vi "Test XYZ Table Stage Module All Axis.vi"() -> ()   [LabVIEW 2018]
uses:
  Hardware Mfg/Thorlabs Translation Stages/Controls/Translation Stage Cluster.ctl
  General/Controls/Translation Stage Types.ctl
  General/Controls/Translation Stage Parameters.ctl
  General/Controls/Set Get Controls.ctl
  Hardware Mfg/Thorlabs Translation Stages/Controls/Motion Translation Module Control2.ctl
panel:
  in  "Table Stages":T1={"X Stage"={"Position"=0.0, "Is.Enabled?"=FALSE, "Is.Connected?"=FALSE, "Device SN"="45876425", "AccelerationMaximum"=0.0, "VelocityMaximum"=0.0, "Acceleration"=0.0, "Velocity"=0.0, "waitTimeout (ms)"=0, "Model"=enum."Thorlabs LTS", "Is.Homed?"=FALSE}, "Y Stage"={"Position"=0.0, "Is.Enabled?"=FALSE, "Is.Connected?"=FALSE, "Device SN"="45995820", "AccelerationMaximum"=0.0, "VelocityMaximum"=0.0, "Acceleration"=0.0, "Velocity"=0.0, "waitTimeout (ms)"=0, "Model"=enum."Thorlabs LTS", "Is.Homed?"=FALSE}, "Z Stage"={"Position"=0.0, "Is.Enabled?"=FALSE, "Is.Connected?"=FALSE, "Device SN"="49107444", "AccelerationMaximum"=0.0, "VelocityMaximum"=0.0, "Acceleration"=0.0, "Velocity"=0.0, "waitTimeout (ms)"=0, "Model"=enum."Thorlabs MLJ", "Is.Homed?"=FALSE}}
  out "Cluster":T4
  in  "Z Pos":dbl caption="Position"
  in  "Y Pos":dbl caption="Position"
  in  "X Pos":dbl caption="Position"
  out "Error Out":errorcluster
  in  "Uninit":bool
  in  "Init":bool
  in  "Cancel Button":bool
  in  "Position":bool
  in  "Stop":bool
  in  "Home":bool
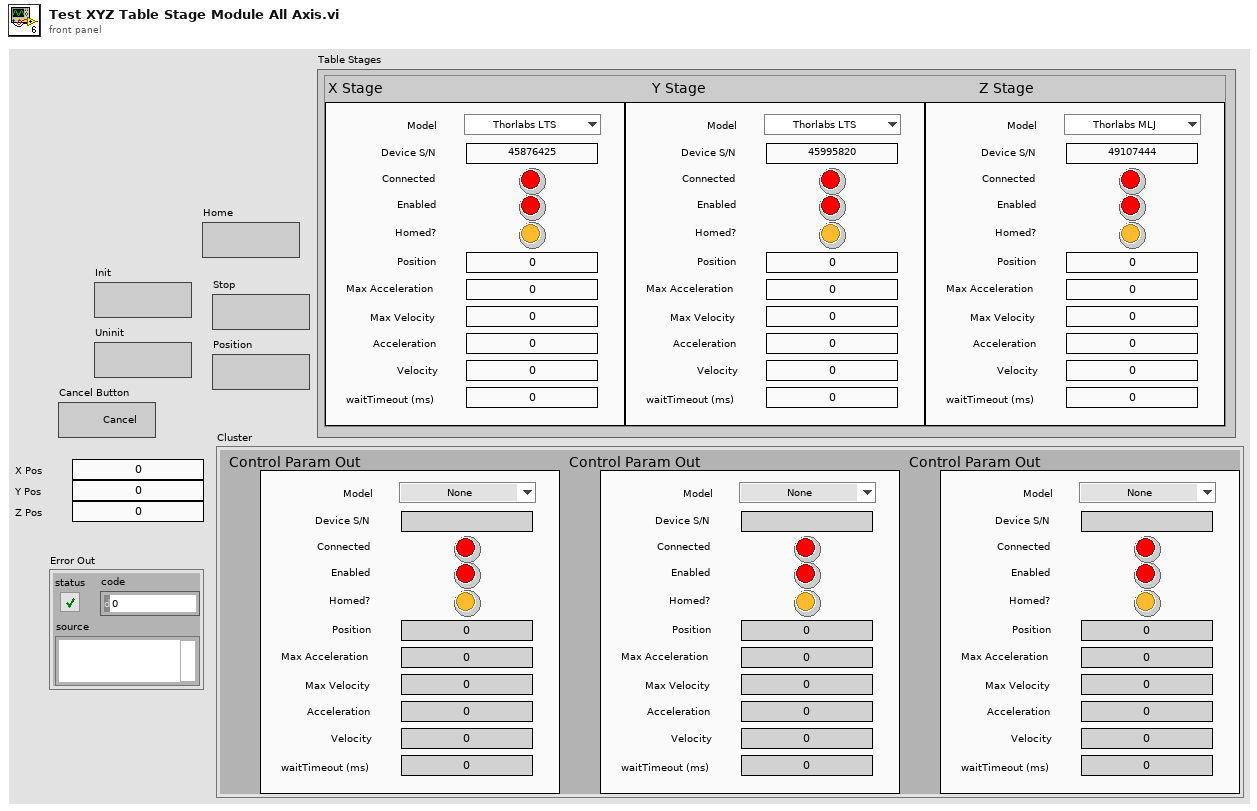
[diagram p1: front panel]
types:
  T1 = typedef "Translation Stage Parameters.ctl" = cluster{"X Stage":T2, "Y Stage":T2, "Z Stage":T2}
  T2 = typedef "Translation Stage Cluster.ctl" = cluster{"Position":dbl, "Is.Enabled?":bool, "Is.Connected?":bool, "Device SN":string, "AccelerationMaximum":dbl, "VelocityMaximum":dbl, "Acceleration":dbl, "Velocity":dbl, "waitTimeout (ms)":i32, "Model":T3, "Is.Homed?":bool}
  T3 = typedef "Translation Stage Types.ctl" = enum16{"None", "Thorlabs LTS", "Thorlabs MLJ"}
  T4 = cluster{"Control Param Out":T2, "Control Param Out":T2, "Control Param Out":T2}
  T5 = typedef "Motion Translation Module Control2.ctl" = enum16{"Init", "Home", "Status", "Velocity/Accel", "Position", "Jog", "Stop", "Uninit", "Enable", "Disable"}
  T6 = typedef "Set Get Controls.ctl" = enum16{"Set", "Get"}
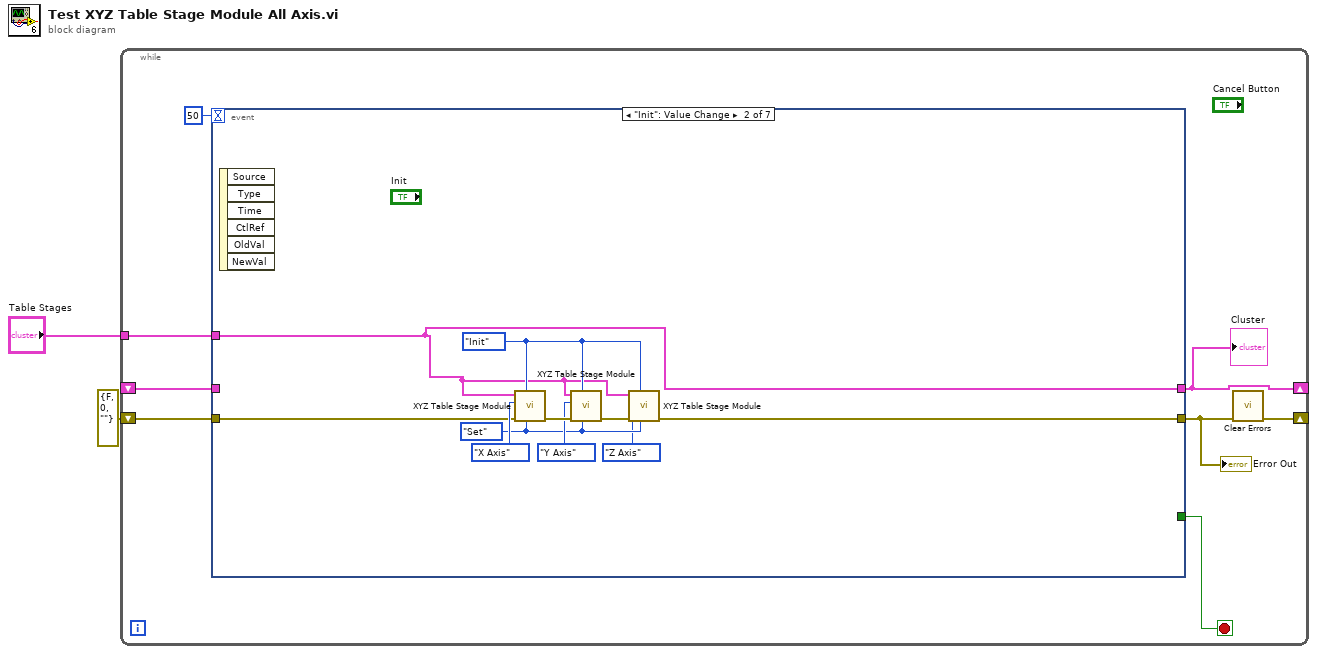
[diagram p0: block diagram]
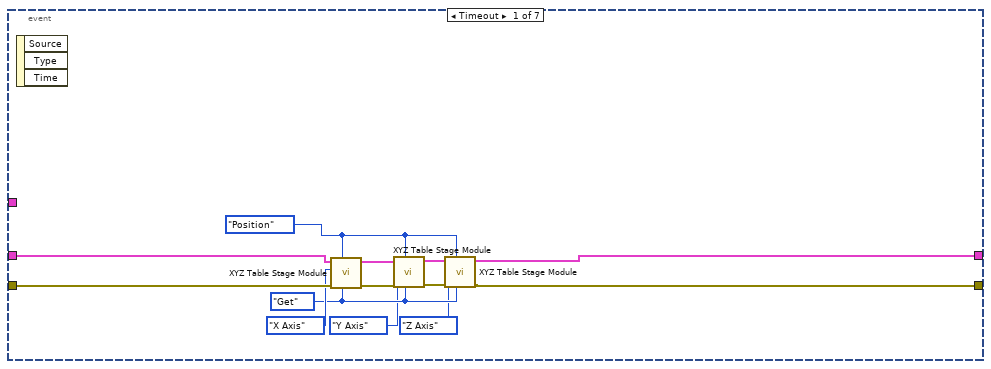
[diagram p2: hidden frame]
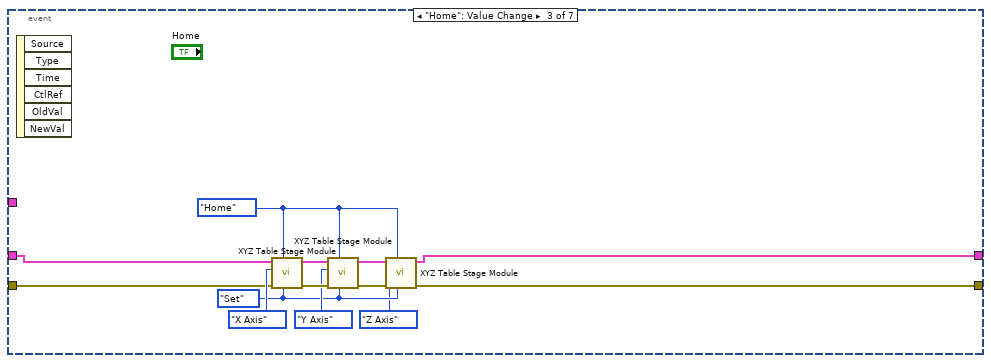
[diagram p3: hidden frame]
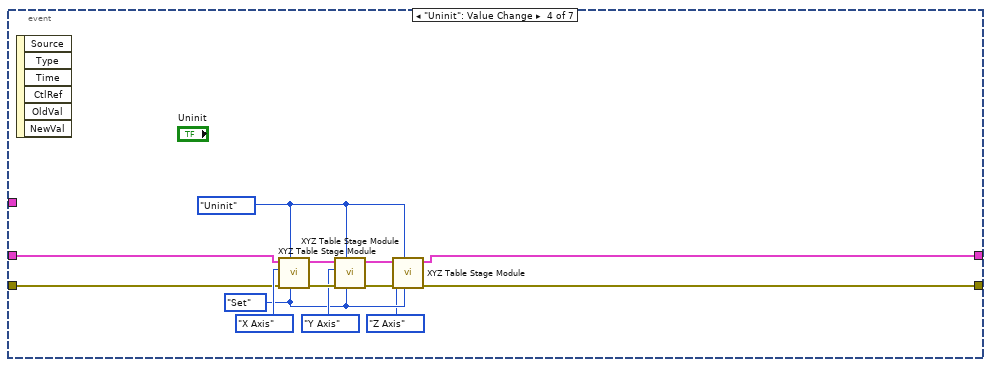
[diagram p4: hidden frame]
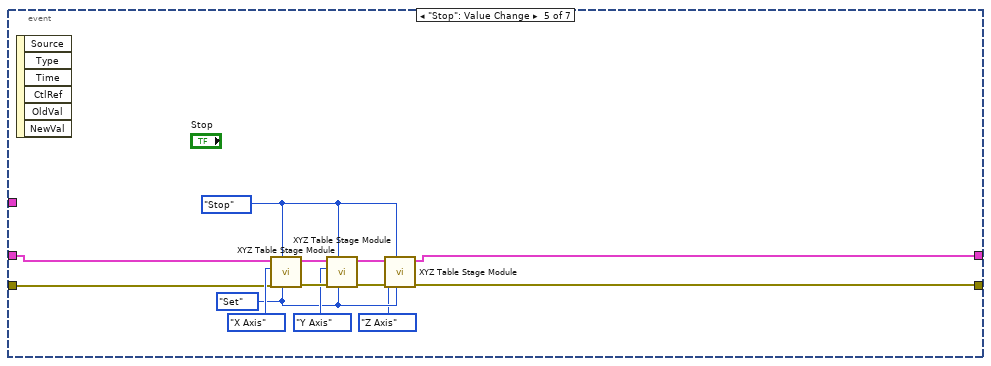
[diagram p5: hidden frame]
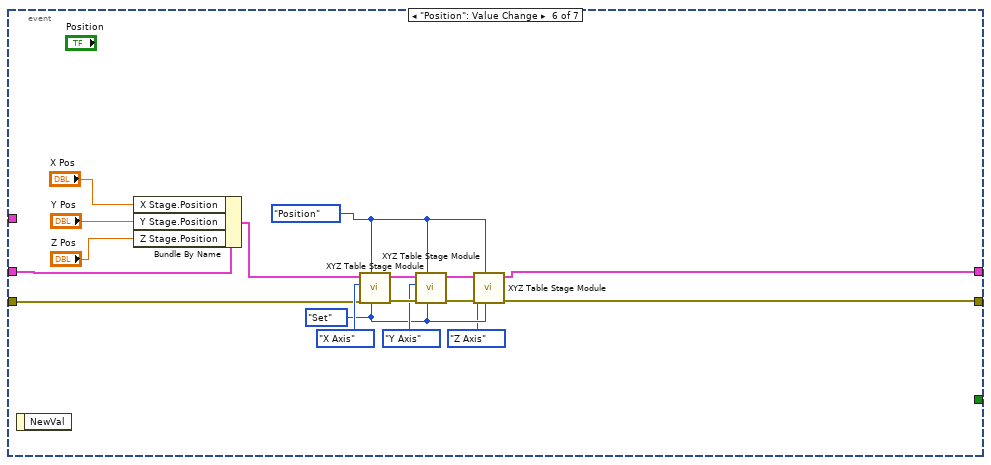
[diagram p6: hidden frame]
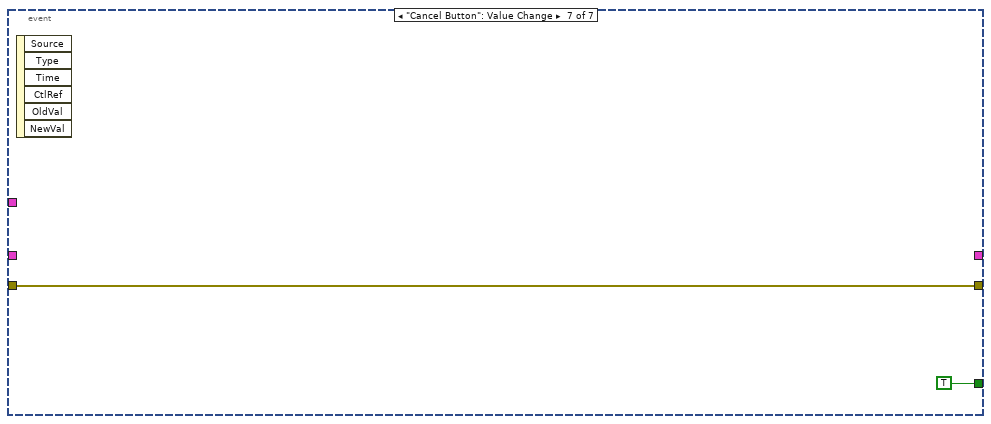
[diagram p7: hidden frame]
diagram:
  n1 = while {
    shift-right: [w5] -> _
    shift-left: errorcluster {"status"=FALSE, "code"=0, "source"=""} ("Error Out") -> [w7]
    shift-right: [w4] -> _
    shift-left: _ -> [w6]
    tunnel: "Table Stages" -> [w3]
    stop <- w9 stop-if-true
    n2 = event shown="[1] \"Init\": Value Change" {
      selector: _ -> [_ _ _ _ _ _ _]
      dyn-events: _ -> [_ _ _ _ _ _ _]
      timeout: 50 -> [_ _ _ _ _ _ _]
      tunnel: [_ _ _ _ _ _ TRUE] -> w9
      tunnel: [w12 w24 w35 w48 w61 w74 _] -> w4
      tunnel: w6 -> [w22 _ w38 w51 w64 w78 _]
      tunnel: [w13 w31 w39 w52 w65 w81 w90] -> w8
      tunnel: w7 -> [w23 w25 w40 w53 w66 w82 w90]
      tunnel: w3 -> [_ w24 _ _ _ _ _]
      event Timeout {
        w11 = Motion_Translation_Module_Control2."Position" ("Action")
        w16 = Set_Get_Controls."Get" ("Set/Get")
        n3 = event-data() -> ()  [unwired: 1 in, 3 out]
        n4 = call "XYZ Table Stage Module.vi"("Set/Get"=w16, "Action"=w11, "Error In"=w23, "Axis"=enum16{"X Axis", "Y Axis", "Z Axis"}."X Axis", "Table Stages"=w22) -> ("Error Out"=w18:errorcluster, "Table Stages [out]"=w17:T1)  [unwired: 5 in]
        n5 = call "XYZ Table Stage Module.vi"("Set/Get"=w16, "Action"=w11, "Error In"=w18, "Axis"=enum16{"X Axis", "Y Axis", "Z Axis"}."Y Axis", "Table Stages"=w17) -> ("Error Out"=w20:errorcluster, "Table Stages [out]"=w19:T1)  [unwired: 5 in]
        n6 = call "XYZ Table Stage Module.vi"("Set/Get"=w16, "Action"=w11, "Error In"=w20, "Axis"=enum16{"X Axis", "Y Axis", "Z Axis"}."Z Axis", "Table Stages"=w19) -> ("Error Out"=w13:errorcluster, "Table Stages [out]"=w12:T1)  [unwired: 5 in]
      }
      event "Init": Value Change {
        w28 = Set_Get_Controls."Set" ("Set/Get")
        w26 = Motion_Translation_Module_Control2."Init" ("Action")
        n7 = event-data() -> ()  [unwired: 1 in, 6 out]
        n8 = call "XYZ Table Stage Module.vi"("Set/Get"=w28, "Action"=w26, "Error In"=w25, "Axis"=enum16{"X Axis", "Y Axis", "Z Axis"}."X Axis", "Table Stages"=w24) -> ("Error Out"=w32:errorcluster)  [unwired: 5 in, 1 out]
        n9 = call "XYZ Table Stage Module.vi"("Set/Get"=w28, "Action"=w26, "Error In"=w32, "Axis"=enum16{"X Axis", "Y Axis", "Z Axis"}."Y Axis", "Table Stages"=w24) -> ("Error Out"=w33:errorcluster)  [unwired: 5 in, 1 out]
        n10 = call "XYZ Table Stage Module.vi"("Set/Get"=w28, "Action"=w26, "Error In"=w33, "Axis"=enum16{"X Axis", "Y Axis", "Z Axis"}."Z Axis", "Table Stages"=w24) -> ("Error Out"=w31:errorcluster)  [unwired: 5 in, 1 out]
      }
      event "Home": Value Change {
        w34 = Motion_Translation_Module_Control2."Home" ("Action")
        w42 = Set_Get_Controls."Set" ("Set/Get")
        n11 = event-data() -> ()  [unwired: 1 in, 6 out]
        n12 = call "XYZ Table Stage Module.vi"("Set/Get"=w42, "Action"=w34, "Error In"=w40, "Axis"=enum16{"X Axis", "Y Axis", "Z Axis"}."X Axis", "Table Stages"=w38) -> ("Error Out"=w45:errorcluster, "Table Stages [out]"=w37:T1)  [unwired: 5 in]
        n13 = call "XYZ Table Stage Module.vi"("Set/Get"=w42, "Action"=w34, "Error In"=w45, "Axis"=enum16{"X Axis", "Y Axis", "Z Axis"}."Y Axis", "Table Stages"=w37) -> ("Error Out"=w46:errorcluster, "Table Stages [out]"=w36:T1)  [unwired: 5 in]
        n14 = call "XYZ Table Stage Module.vi"("Set/Get"=w42, "Action"=w34, "Error In"=w46, "Axis"=enum16{"X Axis", "Y Axis", "Z Axis"}."Z Axis", "Table Stages"=w36) -> ("Error Out"=w39:errorcluster, "Table Stages [out]"=w35:T1)  [unwired: 5 in]
      }
      event "Uninit": Value Change {
        w47 = Motion_Translation_Module_Control2."Uninit" ("Action")
        w55 = Set_Get_Controls."Set" ("Set/Get")
        n15 = event-data() -> ()  [unwired: 1 in, 6 out]
        n16 = call "XYZ Table Stage Module.vi"("Set/Get"=w55, "Action"=w47, "Error In"=w53, "Axis"=enum16{"X Axis", "Y Axis", "Z Axis"}."X Axis", "Table Stages"=w51) -> ("Error Out"=w58:errorcluster, "Table Stages [out]"=w50:T1)  [unwired: 5 in]
        n17 = call "XYZ Table Stage Module.vi"("Set/Get"=w55, "Action"=w47, "Error In"=w58, "Axis"=enum16{"X Axis", "Y Axis", "Z Axis"}."Y Axis", "Table Stages"=w50) -> ("Error Out"=w59:errorcluster, "Table Stages [out]"=w49:T1)  [unwired: 5 in]
        n18 = call "XYZ Table Stage Module.vi"("Set/Get"=w55, "Action"=w47, "Error In"=w59, "Axis"=enum16{"X Axis", "Y Axis", "Z Axis"}."Z Axis", "Table Stages"=w49) -> ("Error Out"=w52:errorcluster, "Table Stages [out]"=w48:T1)  [unwired: 5 in]
      }
      event "Stop": Value Change {
        w60 = Motion_Translation_Module_Control2."Stop" ("Action")
        w68 = Set_Get_Controls."Set" ("Set/Get")
        n19 = event-data() -> ()  [unwired: 1 in, 6 out]
        n20 = call "XYZ Table Stage Module.vi"("Set/Get"=w68, "Action"=w60, "Error In"=w66, "Axis"=enum16{"X Axis", "Y Axis", "Z Axis"}."X Axis", "Table Stages"=w64) -> ("Error Out"=w71:errorcluster, "Table Stages [out]"=w63:T1)  [unwired: 5 in]
        n21 = call "XYZ Table Stage Module.vi"("Set/Get"=w68, "Action"=w60, "Error In"=w71, "Axis"=enum16{"X Axis", "Y Axis", "Z Axis"}."Y Axis", "Table Stages"=w63) -> ("Error Out"=w72:errorcluster, "Table Stages [out]"=w62:T1)  [unwired: 5 in]
        n22 = call "XYZ Table Stage Module.vi"("Set/Get"=w68, "Action"=w60, "Error In"=w72, "Axis"=enum16{"X Axis", "Y Axis", "Z Axis"}."Z Axis", "Table Stages"=w62) -> ("Error Out"=w65:errorcluster, "Table Stages [out]"=w61:T1)  [unwired: 5 in]
      }
      event "Position": Value Change {
        w73 = Motion_Translation_Module_Control2."Position" ("Action")
        w84 = Set_Get_Controls."Set" ("Set/Get")
        n23 = event-data() -> ()  [unwired: 1 in, 1 out]
        n24 = Bundle By Name(cluster=w78, "X Stage.Position"="X Pos", "Y Stage.Position"="Y Pos", "Z Stage.Position"="Z Pos") -> (w77:T1)
        n25 = call "XYZ Table Stage Module.vi"("Set/Get"=w84, "Action"=w73, "Error In"=w82, "Axis"=enum16{"X Axis", "Y Axis", "Z Axis"}."X Axis", "Table Stages"=w77) -> ("Error Out"=w87:errorcluster, "Table Stages [out]"=w76:T1)  [unwired: 5 in]
        n26 = call "XYZ Table Stage Module.vi"("Set/Get"=w84, "Action"=w73, "Error In"=w87, "Axis"=enum16{"X Axis", "Y Axis", "Z Axis"}."Y Axis", "Table Stages"=w76) -> ("Error Out"=w88:errorcluster, "Table Stages [out]"=w75:T1)  [unwired: 5 in]
        n27 = call "XYZ Table Stage Module.vi"("Set/Get"=w84, "Action"=w73, "Error In"=w88, "Axis"=enum16{"X Axis", "Y Axis", "Z Axis"}."Z Axis", "Table Stages"=w75) -> ("Error Out"=w81:errorcluster, "Table Stages [out]"=w74:T1)  [unwired: 5 in]
      }
      event "Cancel Button": Value Change {
        n28 = event-data() -> ()  [unwired: 1 in, 6 out]
      }
    }
    "Error Out" <- w8
    "Cluster" <- w4
    n29 = call <vilib>:"Clear Errors.vi"("error in (no error)"=w8) -> ("error out"=w5:errorcluster)  [unwired: 5 in, 1 out]
  }
